vi "Add New Data to Buffer.vi"(0 "Data Buffer In":sgl[][](array[numeric]), 1 "Scaled Channel Data":sgl[][](array[numeric]), 2 "RMS Data":sgl[][](array[numeric]), 3 "Pk-Pk Data":sgl[][](array[numeric]), 4 "Freq Data":sgl[][](array[numeric]), 7 "# Samples Read":u32, 9 "Data Indexes":i32[](array[numeric])) -> (14 "Data Buffer Out":sgl[][](array[numeric]), 15 "Data Out":sgl[][](array[numeric]))   [LabVIEW 2019]
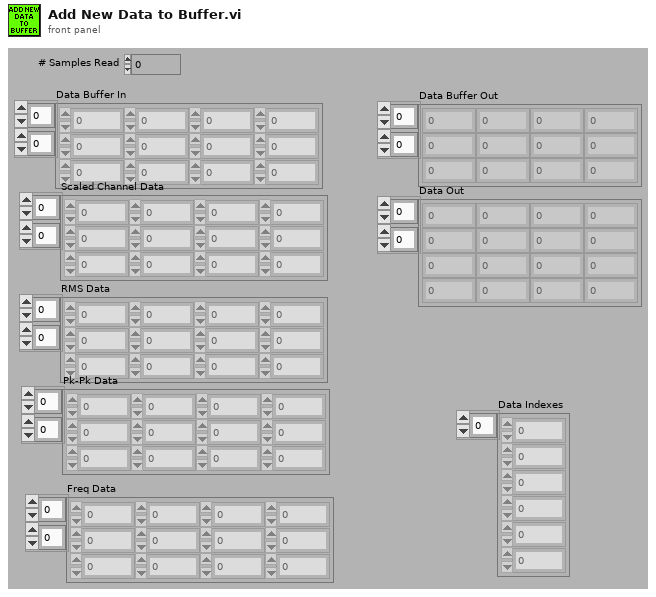
[diagram p1: front panel]
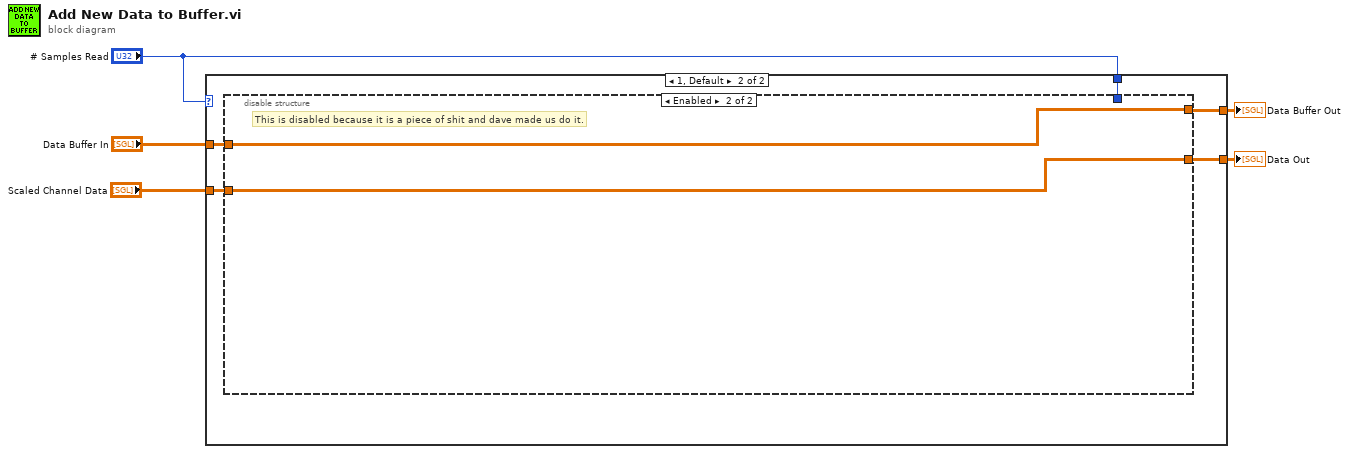
[diagram p0: block diagram]
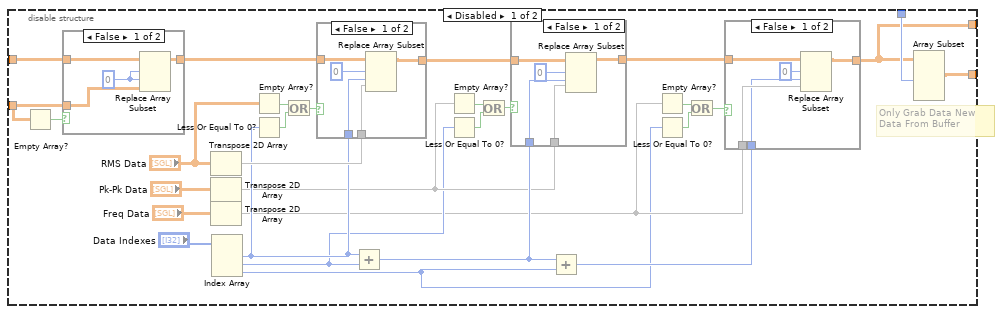
[diagram p3: hidden frame]
diagram:
  n1 = case shown="1, Default" "# Samples Read" {
    tunnel: "Data Buffer In" -> [w7 w12]
    tunnel: "# Samples Read" -> [_ w11]
    tunnel: [w6 w10] -> w4
    tunnel: [w7 w9] -> w3
    tunnel: "Scaled Channel Data" -> [w6 w8]
    frame 0 {
    }
    frame 1, Default {
      n2 = disable-structure shown="Enabled" {
        disable-tunnel: w12 -> [w42 w67]
        disable-tunnel: w11 -> [w41 _]
        disable-tunnel: [w40 w66] -> w10
        disable-tunnel: [w32 w67] -> w9
        disable-tunnel: w8 -> [w13 w66]
        frame Disabled {
          # "Only Grab Data New Data From Buffer"
          n3 = Empty Array?(array=w13) -> (empty?=w14:bool)
          n4 = case shown="False" w14 {
            tunnel: w42 -> [w46 w47]
            tunnel: w13 -> [w45 _]
            tunnel: [w43 w47] -> w36
            frame False {
              w44 = 0 ("disabled index (col)")
              n5 = Replace Array Subset(array=w46, new element=w45, index (row)=w44, index (col)=w44) -> (w43:sgl[][])
            }
            frame True {
            }
          }
          n6 = Transpose 2D Array(2D array="RMS Data") -> (transposed array=w35:sgl[][])
          n7 = Transpose 2D Array(2D array="Pk-Pk Data") -> (transposed array=w21:sgl[][])
          n8 = Transpose 2D Array(2D array="Freq Data") -> (transposed array=w16:sgl[][])
          n9 = Index Array(array="Data Indexes") -> (element #1=w25:i32, element #2=w20:i32, element #3=w15:i32)  [unwired: 3 in]
          n10 = Empty Array?(array="RMS Data") -> (empty?=w28:bool)
          n11 = Less Or Equal To 0?(x=w25) -> (x <= 0?=w26:bool)
          n12 = Or(x=w28, y=w26) -> (x .or. y?=w27:bool)
          n13 = case shown="False" w27 {
            tunnel: w36 -> [w64 w65]
            tunnel: w35 -> [w63 _]
            tunnel: [w62 w65] -> w34
            tunnel: w25 -> [w61 _]
            frame False {
              n14 = Replace Array Subset(array=w64, new element=w63, index (row)=0 ("disabled index (row)"), index (col)=w61) -> (w62:sgl[][])
            }
            frame True {
            }
          }
          n15 = Add(x=w25, y=w20) -> (x+y=w31:i32)
          n16 = Empty Array?(array=w21) -> (empty?=w23:bool)
          n17 = Less Or Equal To 0?(x=w20) -> (x <= 0?=w24:bool)
          n18 = Or(x=w23, y=w24) -> (x .or. y?=w22:bool)
          n19 = case shown="False" w22 {
            tunnel: w34 -> [w58 w59]
            tunnel: [w57 w59] -> w33
            tunnel: w21 -> [w56 _]
            tunnel: w31 -> [w55 _]
            frame False {
              n20 = Replace Array Subset(array=w58, new element=w56, index (row)=0 ("disabled index (row)"), index (col)=w55) -> (w57:sgl[][])
            }
            frame True {
            }
          }
          n21 = Add(x=w31, y=w15) -> (x+y=w30:i32)
          n22 = Empty Array?(array=w16) -> (empty?=w19:bool)
          n23 = Less Or Equal To 0?(x=w15) -> (x <= 0?=w18:bool)
          n24 = Or(x=w19, y=w18) -> (x .or. y?=w17:bool)
          n25 = case shown="False" w17 {
            tunnel: w33 -> [w52 w53]
            tunnel: [w51 w53] -> w32
            tunnel: w16 -> [w50 _]
            tunnel: w30 -> [w49 _]
            frame False {
              n26 = Replace Array Subset(array=w52, new element=w50, index (row)=0 ("disabled index (row)"), index (col)=w49) -> (w51:sgl[][])
            }
            frame True {
            }
          }
          n27 = Array Subset(array=w32, length (row)=w41) -> (w40:sgl[][])  [unwired: 3 in]
        }
        frame Enabled {
          # "This is disabled because it is a piece of shit and dave made us do it."
        }
      }
    }
  }
  "Data Out" <- w4
  "Data Buffer Out" <- w3
